vi "PlotHand.vi"(8 "error in":errorcluster, 11 "Frame":T1={"Id"=1994076, "Timestamp"=867814299078, "CurrentFramesPerSecond"=108.23245, "Hands"=[{"IsLeft"=FALSE, "IsRight"=TRUE, "Id"=373, "FrameId"=1994076, "Confidence"=1.0, "TimeVisible"=42500670.0, "PalmPosition"={"Pitch"=2.5588596, "Yaw"=-2.4626648, "Roll"=-2.2557082, "Magnitude"=877.05, "XYZ"=[-490.0468, 400.27893, 607.32825]}, "Fingers"=[{"IsExtended"=TRUE, "Id"=3730, "Type"=0, "HandId"=373, "Length"=96.07253, "Width"=20.172712, "TimeVisible"=42500670.0, "TipPosition"={"Pitch"=2.4633646, "Yaw"=-2.4019272, "Roll"=-2.2941506, "Magnitude"=882.3877, "XYZ"=[-511.08807, 451.30103, 560.111]}, "Bones"=[{"Type"=0, "Width"=20.172712, "Length"=0.0, "Center"={"Pitch"=2.5631144, "Yaw"=-2.4741964, "Roll"=-2.2627635, "Magnitude"=934.0878, "XYZ"=[-514.43164, 426.28302, 652.8116]}, "Direction"={"Pitch"=3.1415927, "Yaw"=3.1415927, "Roll"=3.1415927, "Magnitude"=0.0, "XYZ"=[0.0, 0.0, 0.0]}, "NextJoint"={"Pitch"=2.5631144, "Yaw"=-2.4741964, "Roll"=-2.2627635, "Magnitude"=934.0878, "XYZ"=[-514.43164, 426.28302, 652.8116]}, "PrevJoint"={"Pitch"=2.5631144, "Yaw"=-2.4741964, "Roll"=-2.2627635, "Magnitude"=934.0878, "XYZ"=[-514.43164, 426.28302, 652.8116]}}, {"Type"=1, "Width"=20.172712, "Length"=46.94757, "Center"={"Pitch"=2.5357366, "Yaw"=-2.4600737, "Roll"=-2.2776248, "Magnitude"=925.0941, "XYZ"=[-513.2206, 438.3053, 632.6865]}, "Direction"={"Pitch"=0.53849036, "Yaw"=0.06010279, "Roll"=3.0411992, "Magnitude"=1.0, "XYZ"=[0.0515907, 0.5121576, -0.85734063]}, "NextJoint"={"Pitch"=2.5076604, "Yaw"=-2.445371, "Roll"=-2.292186, "Magnitude"=916.6135, "XYZ"=[-512.0096, 450.32758, 612.5615]}, "PrevJoint"={"Pitch"=2.5631144, "Yaw"=-2.4741964, "Roll"=-2.2627635, "Magnitude"=934.0878, "XYZ"=[-514.43164, 426.28302, 652.8116]}}, {"Type"=2, "Width"=20.172712, "Length"=32.13855, "Center"={"Pitch"=2.4914145, "Yaw"=-2.4331112, "Roll"=-2.2966583, "Magnitude"=907.74, "XYZ"=[-511.48987, 453.94366, 596.913]}, "Direction"={"Pitch"=0.22709501, "Yaw"=0.033200543, "Roll"=2.9988427, "Magnitude"=1.0, "XYZ"=[0.032343067, 0.22503029, -0.97381485]}, "NextJoint"={"Pitch"=2.4747179, "Yaw"=-2.4204643, "Roll"=-2.3011045, "Magnitude"=899.0661, "XYZ"=[-510.97012, 457.55972, 581.2645]}, "PrevJoint"={"Pitch"=2.5076604, "Yaw"=-2.445371, "Roll"=-2.292186, "Magnitude"=916.6135, "XYZ"=[-512.0096, 450.32758, 612.5615]}}, {"Type"=3, "Width"=20.172712, "Length"=22.06028, "Center"={"Pitch"=2.4691207, "Yaw"=-2.4112904, "Roll"=-2.297638, "Magnitude"=890.6976, "XYZ"=[-511.0291, 454.43036, 570.68774]}, "Direction"={"Pitch"=-0.28766397, "Yaw"=-0.0055758716, "Roll"=-0.018843614, "Magnitude"=0.99999994, "XYZ"=[-0.0053467336, -0.2837089, -0.9588955]}, "NextJoint"={"Pitch"=2.4633646, "Yaw"=-2.4019272, "Roll"=-2.2941506, "Magnitude"=882.3877, "XYZ"=[-511.08807, 451.30103, 560.111]}, "PrevJoint"={"Pitch"=2.4747179, "Yaw"=-2.4204643, "Roll"=-2.3011045, "Magnitude"=899.0661, "XYZ"=[-510.97012, 457.55972, 581.2645]}}]}, {"IsExtended"=TRUE, "Id"=3731, "Type"=1, "HandId"=373, "Length"=75.68024, "Width"=19.268976, "TimeVisible"=42500670.0, "TipPosition"={"Pitch"=2.434744, "Yaw"=-2.3595173, "Roll"=-2.2809286, "Magnitude"=829.2213, "XYZ"=[-499.8062, 429.71277, 503.13885]}, "Bones"=[{"Type"=0, "Width"=19.268976, "Length"=69.1923, "Center"={"Pitch"=2.5401537, "Yaw"=-2.4662747, "Roll"=-2.279225, "Magnitude"=891.7693, "XYZ"=[-491.43066, 421.05786, 613.56226]}, "Direction"={"Pitch"=-0.08703206, "Yaw"=0.03905984, "Roll"=0.42109984, "Magnitude"=1.0, "XYZ"=[0.038902335, -0.08685643, -0.995461]}, "NextJoint"={"Pitch"=2.5163376, "Yaw"=-2.439278, "Roll"=-2.277042, "Magnitude"=866.21875, "XYZ"=[-490.0848, 418.05295, 579.1231]}, "PrevJoint"={"Pitch"=2.562119, "Yaw"=-2.4914331, "Roll"=-2.281388, "Magnitude"=917.91266, "XYZ"=[-492.77655, 424.06274, 648.00134]}}, {"Type"=1, "Width"=19.268976, "Length"=40.49642, "Center"={"Pitch"=2.4949355, "Yaw"=-2.4226556, "Roll"=-2.2825632, "Magnitude"=854.8512, "XYZ"=[-489.51468, 422.25812, 559.3246]}, "Direction"={"Pitch"=0.20928793, "Yaw"=0.028788606, "Roll"=3.0068362, "Magnitude"=1.0, "XYZ"=[0.028157026, 0.20768104, -0.97779125]}, "NextJoint"={"Pitch"=2.472708, "Yaw"=-2.4053361, "Roll"=-2.2880452, "Magnitude"=843.8164, "XYZ"=[-488.94455, 426.4633, 539.52606]}, "PrevJoint"={"Pitch"=2.5163376, "Yaw"=-2.439278, "Roll"=-2.277042, "Magnitude"=866.21875, "XYZ"=[-490.0848, 418.05295, 579.1231]}}, {"Type"=2, "Width"=19.268976, "Length"=22.783022, "Center"={"Pitch"=2.460581, "Yaw"=-2.3933928, "Roll"=-2.2884817, "Magnitude"=838.4589, "XYZ"=[-490.44525, 428.1495, 528.3605]}, "Direction"={"Pitch"=0.14988618, "Yaw"=-0.13360453, "Roll"=-2.4143357, "Magnitude"=1.0, "XYZ"=[-0.13173996, 0.14802411, -0.98017013]}, "NextJoint"={"Pitch"=2.4481795, "Yaw"=-2.3812094, "Roll"=-2.2889156, "Magnitude"=833.2227, "XYZ"=[-491.94598, 429.83572, 517.1948]}, "PrevJoint"={"Pitch"=2.472708, "Yaw"=-2.4053361, "Roll"=-2.2880452, "Magnitude"=843.8164, "XYZ"=[-488.94455, 426.4633, 539.52606]}}, {"Type"=3, "Width"=19.268976, "Length"=16.104925, "Center"={"Pitch"=2.4415162, "Yaw"=-2.3703985, "Roll"=-2.2849042, "Magnitude"=831.1854, "XYZ"=[-495.8761, 429.77423, 510.16684]}, "Direction"={"Pitch"=-0.008747329, "Yaw"=-0.5098862, "Roll"=-1.5551549, "Magnitude"=1.0, "XYZ"=[-0.48806372, -0.007634641, -0.8727746]}, "NextJoint"={"Pitch"=2.434744, "Yaw"=-2.3595173, "Roll"=-2.2809286, "Magnitude"=829.2213, "XYZ"=[-499.8062, 429.71277, 503.13885]}, "PrevJoint"={"Pitch"=2.4481795, "Yaw"=-2.3812094, "Roll"=-2.2889156, "Magnitude"=833.2227, "XYZ"=[-491.94598, 429.83572, 517.1948]}}]}, {"IsExtended"=TRUE, "Id"=3732, "Type"=2, "HandId"=373, "Length"=85.8772, "Width"=18.924694, "TimeVisible"=42500670.0, "TipPosition"={"Pitch"=2.4867768, "Yaw"=-2.37957, "Roll"=-2.2483323, "Magnitude"=786.44617, "XYZ"=[-474.64014, 381.8927, 497.36536]}, "Bones"=[{"Type"=0, "Width"=18.924694, "Length"=65.61695, "Center"={"Pitch"=2.5583334, "Yaw"=-2.4756398, "Roll"=-2.269351, "Magnitude"=883.4468, "XYZ"=[-484.472, 406.86963, 616.6216]}, "Direction"={"Pitch"=-0.21661115, "Yaw"=0.08708795, "Roll"=0.37769556, "Magnitude"=0.99999994, "XYZ"=[0.0849602, -0.21414411, -0.9731002]}, "NextJoint"={"Pitch"=2.5417883, "Yaw"=-2.4524946, "Roll"=-2.2636204, "Magnitude"=856.6004, "XYZ"=[-481.68457, 399.8439, 584.6957]}, "PrevJoint"={"Pitch"=2.573566, "Yaw"=-2.4972546, "Roll"=-2.2749624, "Magnitude"=910.68384, "XYZ"=[-487.2594, 413.8954, 648.54755]}}, {"Type"=1, "Width"=18.924694, "Length"=45.4337, "Center"={"Pitch"=2.5286622, "Yaw"=-2.4379056, "Roll"=-2.2628262, "Magnitude"=837.4656, "XYZ"=[-477.543, 395.76584, 562.735]}, "Direction"={"Pitch"=-0.1836069, "Yaw"=0.18640089, "Roll"=0.79312426, "Magnitude"=1.0, "XYZ"=[0.18231273, -0.17951714, -0.96671385]}, "NextJoint"={"Pitch"=2.5147374, "Yaw"=-2.4225283, "Roll"=-2.262017, "Magnitude"=818.5139, "XYZ"=[-473.40143, 391.68777, 540.7743]}, "PrevJoint"={"Pitch"=2.5417883, "Yaw"=-2.4524946, "Roll"=-2.2636204, "Magnitude"=856.6004, "XYZ"=[-481.68457, 399.8439, 584.6957]}}, {"Type"=2, "Width"=18.924694, "Length"=26.804226, "Center"={"Pitch"=2.506685, "Yaw"=-2.4099944, "Roll"=-2.257922, "Magnitude"=808.73584, "XYZ"=[-473.77435, 388.73895, 527.70593]}, "Direction"={"Pitch"=-0.22192916, "Yaw"=-0.028528724, "Roll"=-0.12579787, "Magnitude"=1.0, "XYZ"=[-0.027825821, -0.22002666, -0.97509694]}, "NextJoint"={"Pitch"=2.4983253, "Yaw"=-2.3971212, "Roll"=-2.2538054, "Magnitude"=799.06287, "XYZ"=[-474.14728, 385.79013, 514.6376]}, "PrevJoint"={"Pitch"=2.5147374, "Yaw"=-2.4225283, "Roll"=-2.262017, "Magnitude"=818.5139, "XYZ"=[-473.40143, 391.68777, 540.7743]}}, {"Type"=3, "Width"=18.924694, "Length"=17.713339, "Center"={"Pitch"=2.4926243, "Yaw"=-2.3884232, "Roll"=-2.2510736, "Magnitude"=792.73016, "XYZ"=[-474.3937, 383.84143, 506.00146]}, "Direction"={"Pitch"=-0.22193053, "Yaw"=-0.028527038, "Roll"=-0.1257897, "Magnitude"=1.0, "XYZ"=[-0.027824167, -0.220028, -0.97509664]}, "NextJoint"={"Pitch"=2.4867768, "Yaw"=-2.37957, "Roll"=-2.2483323, "Magnitude"=786.44617, "XYZ"=[-474.64014, 381.8927, 497.36536]}, "PrevJoint"={"Pitch"=2.4983253, "Yaw"=-2.3971212, "Roll"=-2.2538054, "Magnitude"=799.06287, "XYZ"=[-474.14728, 385.79013, 514.6376]}}]}, {"IsExtended"=TRUE, "Id"=3733, "Type"=3, "HandId"=373, "Length"=81.787834, "Width"=18.008047, "TimeVisible"=42500670.0, "TipPosition"={"Pitch"=2.5342546, "Yaw"=-2.4019299, "Roll"=-2.221698, "Magnitude"=782.20404, "XYZ"=[-469.03964, 357.23376, 514.0321]}, "Bones"=[{"Type"=0, "Width"=18.008047, "Length"=58.913082, "Center"={"Pitch"=2.5794244, "Yaw"=-2.4847152, "Roll"=-2.2557976, "Magnitude"=879.34296, "XYZ"=[-480.49426, 392.54797, 623.11743]}, "Direction"={"Pitch"=-0.36144292, "Yaw"=0.14001572, "Roll"=0.3568416, "Magnitude"=0.99999994, "XYZ"=[0.1307007, -0.35059085, -0.92736363]}, "NextJoint"={"Pitch"=2.5711985, "Yaw"=-2.4668477, "Roll"=-2.2466943, "Magnitude"=853.3819, "XYZ"=[-476.6443, 382.22076, 595.8005]}, "PrevJoint"={"Pitch"=2.5870347, "Yaw"=-2.5015259, "Roll"=-2.264626, "Magnitude"=905.5178, "XYZ"=[-484.34427, 402.87515, 650.4343]}}, {"Type"=1, "Width"=18.008047, "Length"=42.115032, "Center"={"Pitch"=2.5629508, "Yaw"=-2.4520075, "Roll"=-2.240726, "Magnitude"=835.66595, "XYZ"=[-474.77875, 376.09106, 575.74146]}, "Direction"={"Pitch"=-0.29657066, "Yaw"=0.092735626, "Roll"=0.29543766, "Magnitude"=1.0, "XYZ"=[0.088592574, -0.2910932, -0.9525839]}, "NextJoint"={"Pitch"=2.5542052, "Yaw"=-2.4364896, "Roll"=-2.2346528, "Magnitude"=818.10834, "XYZ"=[-472.9132, 369.96136, 555.6824]}, "PrevJoint"={"Pitch"=2.5711985, "Yaw"=-2.4668477, "Roll"=-2.2466943, "Magnitude"=853.3819, "XYZ"=[-476.6443, 382.22076, 595.8005]}}, {"Type"=2, "Width"=18.008047, "Length"=26.1119, "Center"={"Pitch"=2.5485132, "Yaw"=-2.4265108, "Roll"=-2.2308338, "Magnitude"=807.30646, "XYZ"=[-471.75653, 366.1609, 543.2455]}, "Direction"={"Pitch"=-0.29657012, "Yaw"=0.09273575, "Roll"=0.2954386, "Magnitude"=0.99999994, "XYZ"=[0.08859271, -0.29109266, -0.952584]}, "NextJoint"={"Pitch"=2.542601, "Yaw"=-2.4162462, "Roll"=-2.226973, "Magnitude"=796.5721, "XYZ"=[-470.59988, 362.36038, 530.8086]}, "PrevJoint"={"Pitch"=2.5542052, "Yaw"=-2.4364896, "Roll"=-2.2346528, "Magnitude"=818.10834, "XYZ"=[-472.9132, 369.96136, 555.6824]}}, {"Type"=3, "Width"=18.008047, "Length"=17.611563, "Center"={"Pitch"=2.538483, "Yaw"=-2.4091568, "Roll"=-2.2243452, "Magnitude"=789.37164, "XYZ"=[-469.81976, 359.79706, 522.42035]}, "Direction"={"Pitch"=-0.2965713, "Yaw"=0.09273493, "Roll"=0.29543492, "Magnitude"=1.0, "XYZ"=[0.088591896, -0.29109383, -0.9525838]}, "NextJoint"={"Pitch"=2.5342546, "Yaw"=-2.4019299, "Roll"=-2.221698, "Magnitude"=782.20404, "XYZ"=[-469.03964, 357.23376, 514.0321]}, "PrevJoint"={"Pitch"=2.542601, "Yaw"=-2.4162462, "Roll"=-2.226973, "Magnitude"=796.5721, "XYZ"=[-470.59988, 362.36038, 530.8086]}}]}, {"IsExtended"=TRUE, "Id"=3734, "Type"=4, "HandId"=373, "Length"=64.276276, "Width"=15.996155, "TimeVisible"=42500670.0, "TipPosition"={"Pitch"=2.572578, "Yaw"=-2.4264255, "Roll"=-2.205519, "Magnitude"=807.0307, "XYZ"=[-476.5555, 350.92258, 548.6773]}, "Bones"=[{"Type"=0, "Width"=15.996155, "Length"=54.535183, "Center"={"Pitch"=2.6016126, "Yaw"=-2.4889584, "Roll"=-2.2358158, "Magnitude"=879.3618, "XYZ"=[-482.1407, 378.08466, 630.76904]}, "Direction"={"Pitch"=-0.48648062, "Yaw"=0.23622777, "Roll"=0.4271352, "Magnitude"=1.0, "XYZ"=[0.20813438, -0.4572792, -0.8646247]}, "NextJoint"={"Pitch"=2.5996003, "Yaw"=-2.4762497, "Roll"=-2.2253094, "Magnitude"=854.0358, "XYZ"=[-476.46536, 365.61575, 607.1928]}, "PrevJoint"={"Pitch"=2.603484, "Yaw"=-2.500976, "Roll"=-2.245913, "Magnitude"=904.80066, "XYZ"=[-487.816, 390.55356, 654.3453]}}, {"Type"=1, "Width"=15.996155, "Length"=33.3296, "Center"={"Pitch"=2.5939026, "Yaw"=-2.472801, "Roll"=-2.2280931, "Magnitude"=837.9208, "XYZ"=[-468.64758, 361.69397, 593.0077]}, "Direction"={"Pitch"=-0.2697349, "Yaw"=0.503706, "Roll"=1.1058278, "Magnitude"=1.0, "XYZ"=[0.4691184, -0.23533428, -0.8512025]}, "NextJoint"={"Pitch"=2.587968, "Yaw"=-2.4692035, "Roll"=-2.2309587, "Magnitude"=821.82764, "XYZ"=[-460.82983, 357.77216, 578.8226]}, "PrevJoint"={"Pitch"=2.5996003, "Yaw"=-2.4762497, "Roll"=-2.2253094, "Magnitude"=854.0358, "XYZ"=[-476.46536, 365.61575, 607.1928]}}, {"Type"=2, "Width"=15.996155, "Length"=18.43616, "Center"={"Pitch"=2.584008, "Yaw"=-2.457984, "Roll"=-2.2241263, "Magnitude"=817.7775, "XYZ"=[-465.00934, 355.95172, 570.81067]}, "Direction"={"Pitch"=-0.22342475, "Yaw"=-0.4808281, "Roll"=-1.1600116, "Magnitude"=1.0, "XYZ"=[-0.4534046, -0.19748689, -0.8691509]}, "NextJoint"={"Pitch"=2.5799556, "Yaw"=-2.4466553, "Roll"=-2.2173455, "Magnitude"=813.81177, "XYZ"=[-469.18887, 354.13126, 562.79877]}, "PrevJoint"={"Pitch"=2.587968, "Yaw"=-2.4692035, "Roll"=-2.2309587, "Magnitude"=821.82764, "XYZ"=[-460.82983, 357.77216, 578.8226]}}, {"Type"=3, "Width"=15.996155, "Length"=16.24742, "Center"={"Pitch"=2.5763052, "Yaw"=-2.4365819, "Roll"=-2.2114122, "Magnitude"=810.38763, "XYZ"=[-472.8722, 352.52692, 555.73804]}, "Direction"={"Pitch"=-0.22342654, "Yaw"=-0.48082718, "Roll"=-1.1600078, "Magnitude"=0.99999994, "XYZ"=[-0.4534036, -0.19748855, -0.86915094]}, "NextJoint"={"Pitch"=2.572578, "Yaw"=-2.4264255, "Roll"=-2.205519, "Magnitude"=807.0307, "XYZ"=[-476.5555, 350.92258, 548.6773]}, "PrevJoint"={"Pitch"=2.5799556, "Yaw"=-2.4466553, "Roll"=-2.2173455, "Magnitude"=813.81177, "XYZ"=[-469.18887, 354.13126, 562.79877]}}]}]}]}) -> (0 "error out":errorcluster, 3 "Data to plot":cluster{"Array":sgl[], "Array":sgl[]}[](array[cluster]))   [LabVIEW 2017, in "LeapMotion.lvlib"]
uses:
  LeapMotion.lvlib
  TypeDefs/LEAPframe.ctl
  TypeDefs/LEAPhand.ctl
  TypeDefs/LEAPvector.ctl
  TypeDefs/LEAPfinger.ctl
  TypeDefs/LEAPbone.ctl
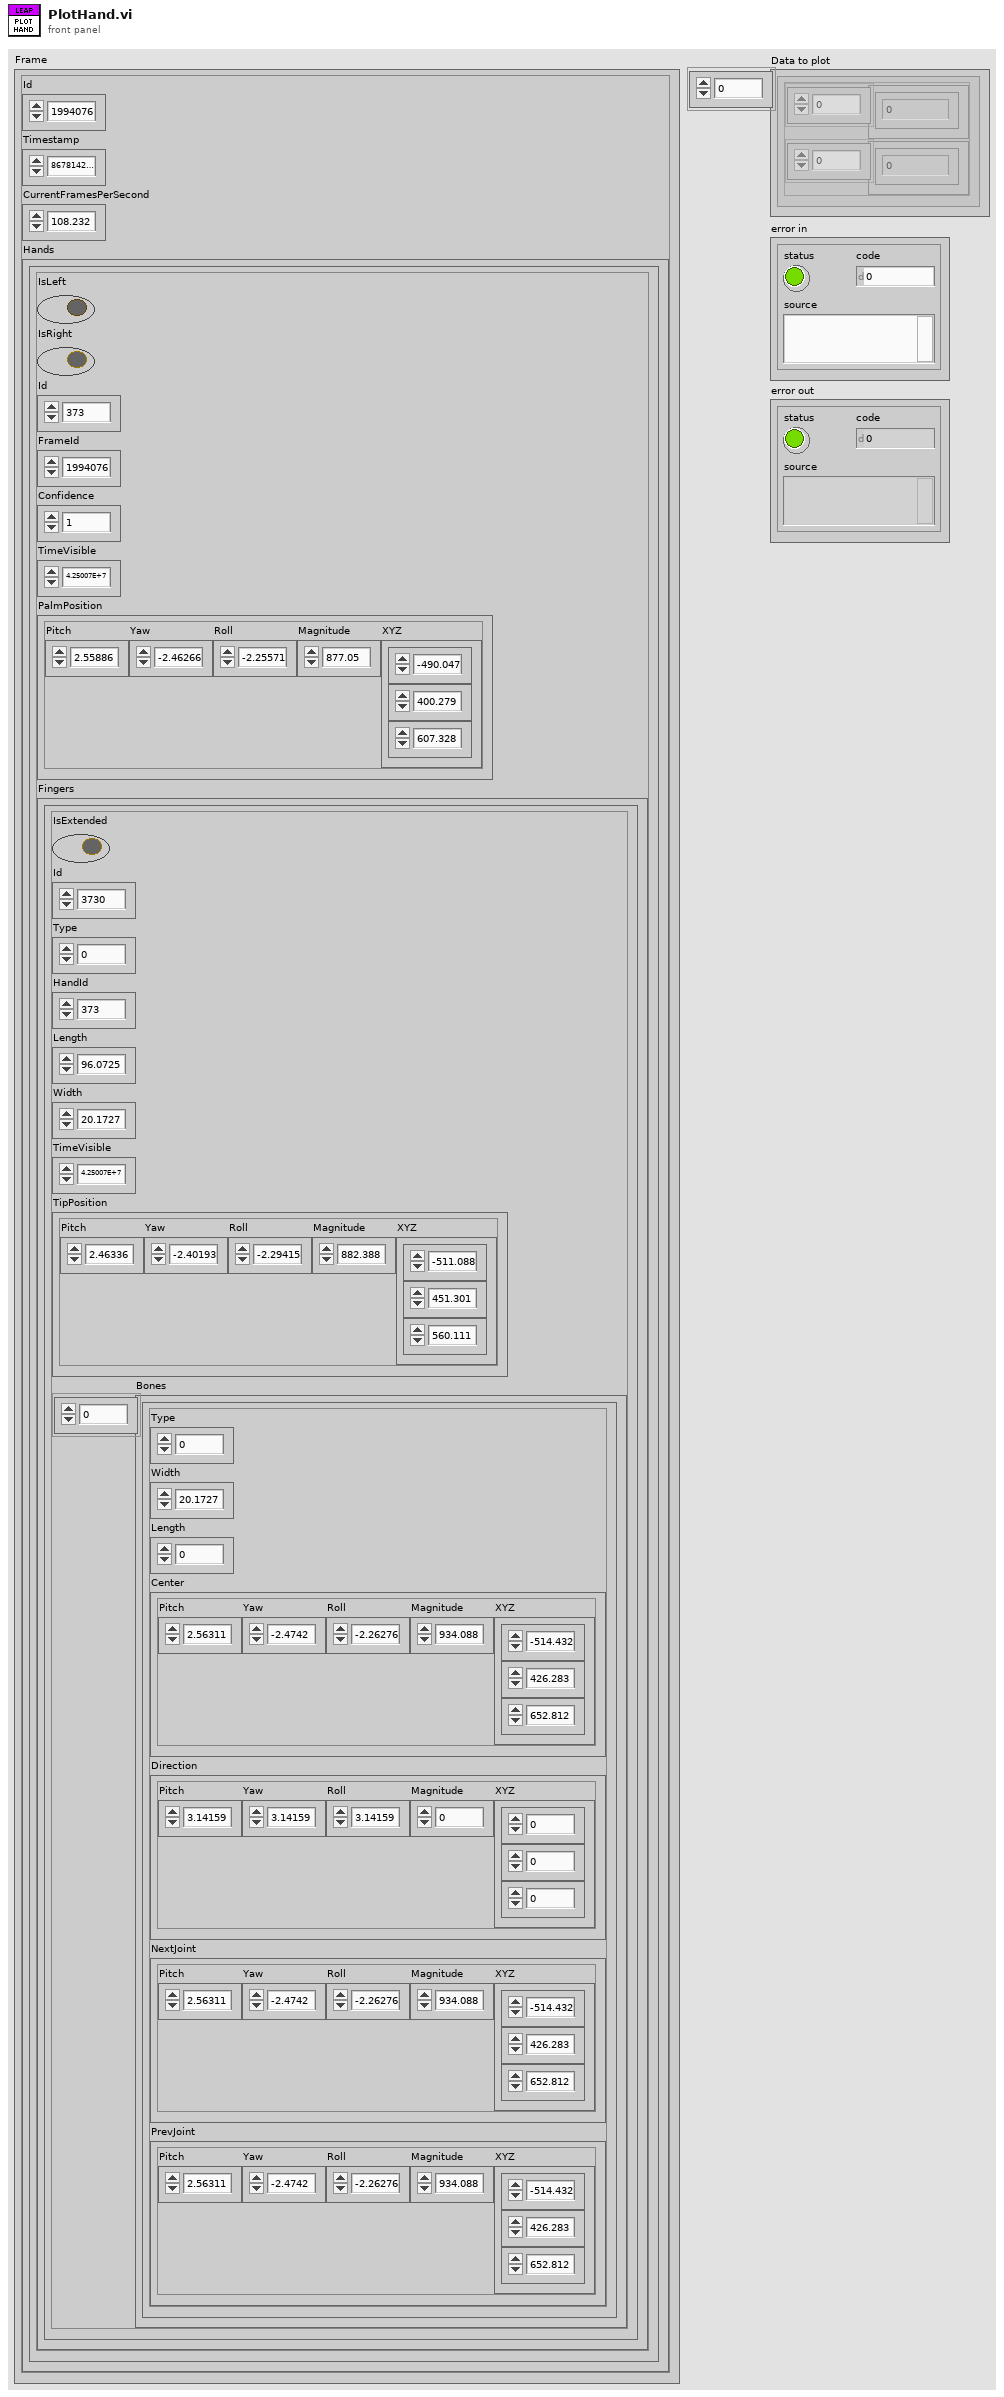
[diagram p1: front panel]
types:
  T1 = typedef "LeapMotion.lvlib/LEAPframe.ctl" = cluster{"Id":i64, "Timestamp":i64, "CurrentFramesPerSecond":sgl, "Hands":T2[]}
  T2 = typedef "LeapMotion.lvlib/LEAPhand.ctl" = cluster{"IsLeft":bool, "IsRight":bool, "Id":i32, "FrameId":i64, "Confidence":sgl, "TimeVisible":sgl, "PalmPosition":T3, "Fingers":T4[]}
  T3 = typedef "LeapMotion.lvlib/LEAPvector.ctl" = cluster{"Pitch":sgl, "Yaw":sgl, "Roll":sgl, "Magnitude":sgl, "XYZ":sgl[]}
  T4 = typedef "LeapMotion.lvlib/LEAPfinger.ctl" = cluster{"IsExtended":bool, "Id":i32, "Type":i32, "HandId":i32, "Length":sgl, "Width":sgl, "TimeVisible":sgl, "TipPosition":T3, "Bones":T5[]}
  T5 = typedef "LeapMotion.lvlib/LEAPbone.ctl" = cluster{"Type":i32, "Width":sgl, "Length":sgl, "Center":T3, "Direction":T3, "NextJoint":T3, "PrevJoint":T3}
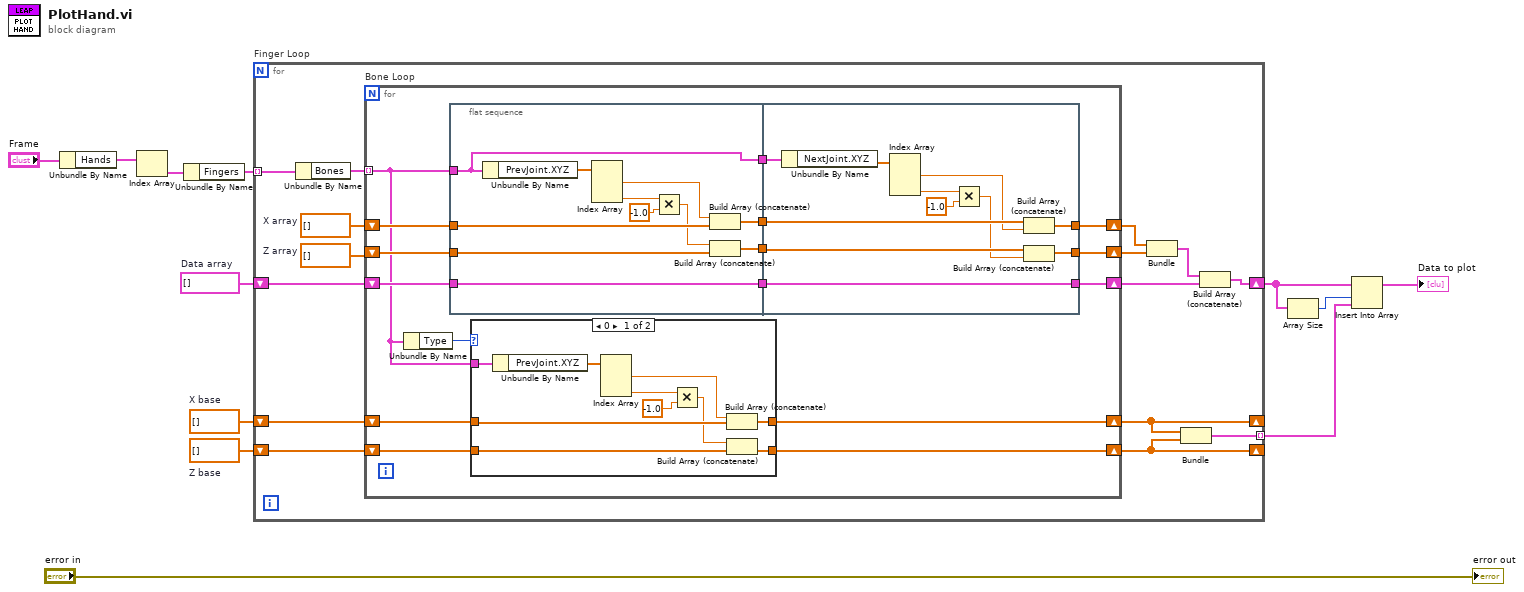
[diagram p0: block diagram]
diagram:
  w4 = sgl[] []  # Z base
  w5 = sgl[] []  # X base
  w8 = cluster{sgl[], sgl[]}[] []  # Data array
  n1 = Unbundle By Name("Frame") -> ("Hands"=w2:T2[])
  n2 = Index Array(array=w2) -> (element=w1:T2)  [unwired: 1 in]
  n3 = Unbundle By Name(w1) -> ("Fingers"=w9:T4[])
  n4 = for "Finger Loop" {
    tunnel: w9 -> [w14] mode=indexing
    shift-right: [w13] -> w3
    shift-left: w8 -> [w23]
    tunnel: [w20] -> w7 mode=indexing
    shift-right: [w17] -> _
    shift-left: w5 -> [w19]
    shift-right: [w16] -> _
    shift-left: w4 -> [w18]
    w24 = sgl[] []  # Z array
    w25 = sgl[] []  # X array
    # "Finger Loop"
    n5 = Unbundle By Name(w14) -> ("Bones"=w26:T5[])
    n6 = for "Bone Loop" {
      tunnel: w26 -> [w32] mode=indexing
      shift-right: [w42] -> w27
      shift-left: w25 -> [w43]
      shift-right: [w40] -> w15
      shift-left: w24 -> [w41]
      shift-right: [w34] -> w21
      shift-left: w23 -> [w36]
      shift-right: [w28] -> w17
      shift-left: w19 -> [w30]
      shift-right: [w29] -> w16
      shift-left: w18 -> [w31]
      # "Bone Loop"
      n7 = Unbundle By Name(w32) -> ("Type"=w33:i32)
      n8 = flat-sequence {
        tunnel: w43 -> [w60]
        tunnel: w32 -> [w59]
        tunnel: [w66] -> w39
        tunnel: w41 -> [w65]
        tunnel: [w64] -> w38
        tunnel: [w59] -> w37
        tunnel: w36 -> [w63]
        tunnel: [w63] -> w35
        tunnel: [w76] -> w42
        tunnel: w39 -> [w77]
        tunnel: [w75] -> w40
        tunnel: w38 -> [w70]
        tunnel: w37 -> [w74]
        tunnel: w35 -> [w73]
        tunnel: [w73] -> w34
        frame #0 {
          n9 = Unbundle By Name(w59) -> ("PrevJoint.XYZ"=w62:sgl[])
          n10 = Index Array(array=w62) -> (element #1=w61:sgl, element #3=w58:sgl)  [unwired: 3 in, 1 out]
          n11 = Multiply(x=w58, y=sgl -1.0) -> (x*y=w57:sgl)
          n12 = Build Array (concatenate)(w61, w60) -> (w66:sgl[])
          n13 = Build Array (concatenate)(w57, w65) -> (w64:sgl[])
        }
        frame #1 {
          n14 = Unbundle By Name(w74) -> ("NextJoint.XYZ"=w72:sgl[])
          n15 = Index Array(array=w72) -> (element #1=w71:sgl, element #3=w67:sgl)  [unwired: 3 in, 1 out]
          n16 = Multiply(x=w67, y=sgl -1.0) -> (x*y=w68:sgl)
          n17 = Build Array (concatenate)(w77, w71) -> (w76:sgl[])
          n18 = Build Array (concatenate)(w70, w68) -> (w75:sgl[])
        }
      }
      n19 = case shown="0" w33 {
        tunnel: w32 -> [w47 _]
        tunnel: w31 -> [w52 w55]
        tunnel: w30 -> [w49 w54]
        tunnel: [w51 w55] -> w29
        tunnel: [w48 w54] -> w28
        frame 0 {
          n20 = Unbundle By Name(w47) -> ("PrevJoint.XYZ"=w53:sgl[])
          n21 = Index Array(array=w53) -> (element #1=w50:sgl, element #3=w45:sgl)  [unwired: 3 in, 1 out]
          n22 = Multiply(x=w45, y=sgl -1.0) -> (x*y=w44:sgl)
          n23 = Build Array (concatenate)(w50, w49) -> (w48:sgl[])
          n24 = Build Array (concatenate)(w44, w52) -> (w51:sgl[])
        }
        frame 1, Default {
        }
      }
    }
    n25 = Bundle("X array"=w27, "Z array"=w15) -> (w22:cluster{"X array":sgl[], "Z array":sgl[]})  [unwired: 1 in]
    n26 = Bundle("X base"=w17, "Z base"=w16) -> (w20:cluster{"X base":sgl[], "Z base":sgl[]})  [unwired: 1 in]
    n27 = Build Array (concatenate)(w22, w21) -> (w13:cluster{"X array":sgl[], "Z array":sgl[]}[])
  }
  n28 = Array Size(array=w3) -> (size(s)=w6:i32)
  n29 = Insert Into Array(array=w3, index=w6, new element=w7) -> (→"Data to plot":cluster{sgl[], sgl[]}[])
  "error out" <- "error in"
